vi "lib Match Pattern 1d array.vi"(8 "error in (no error)":errorcluster, 10 "Search Pattern":string, 11 "Array":string[](array[string])) -> (0 "error out":errorcluster, 2 "match str":string, 3 "index":i32)   [LabVIEW 2016]
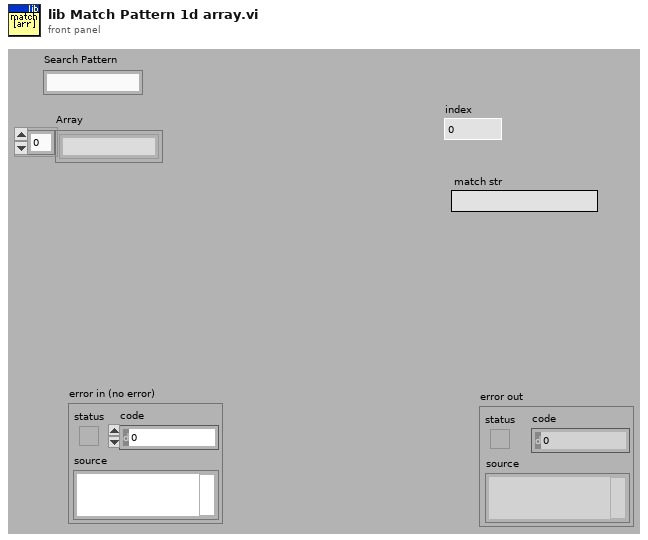
[diagram p1: front panel]
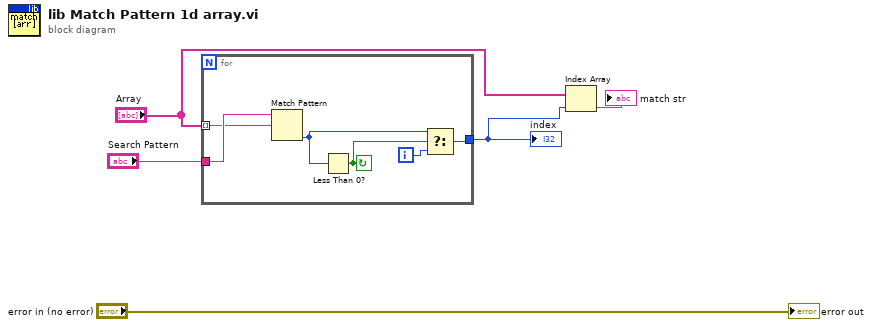
[diagram p0: block diagram]
diagram:
  n1 = for {
    tunnel: "Array" -> [w6] mode=indexing
    tunnel: "Search Pattern" -> [w7]
    tunnel: [w11] -> w2
    i -> [w9]
    stop <- w10 continue-if-true
    n2 = Match Pattern(string=w7, regular expression=w6) -> (offset past match=w8:i32)  [unwired: 1 in, 3 out]
    n3 = Less Than 0?(x=w8) -> (x < 0?=w10:bool)
    n4 = Select(t=w8, s=w10, f=w9) -> (s? t:f=w11:i32)
  }
  "index" <- w2
  n5 = Index Array(array="Array", index=w2) -> (element=→"match str":string)
  "error out" <- "error in (no error)"
